vi "FPGA_PPG_reset.vi"(0 "resource_in":refnum<visa-resource-name>, 5 "error in (no error)":errorcluster) -> (14 "resource_out":refnum<visa-resource-name>, 19 "error out":errorcluster)   [LabVIEW 2014, in "NI-FPGA_PPG_Driver.lvlib"]
doc: "Resets the FPGA to default state (uninitialised).\n\nContact: Falk Ziegler, eMail: ziegler@physik.uni-greifswald.de"
uses:
  NI-FPGA_PPG_Driver.lvlib
  <vilib>/rvi/interface/nirviReadWriteControl/nirviReadWriteControl.xnode
  target/FPGA_target_state_type.ctl
  FPGA_PPG_action_type.ctl
  <vilib>/rvi/errors/niLvFpgaAdjustHostInterfaceError.vi
  FPGA_PPG_vi_ref.ctl
  FPGA Bitfiles/TiTaProj_COF_PPG_100MHz.lvbitx
  <vilib>/rvi/errors/niLvFpgaMergeErrorWithErrorCode.vi
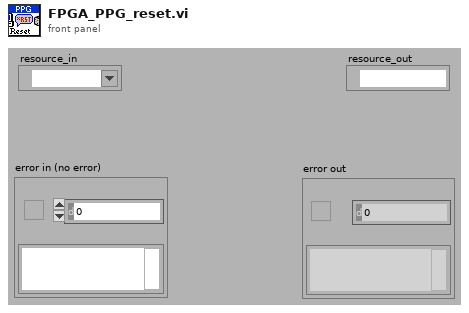
[diagram p1: front panel]
types:
  T1 = typedef "NI-FPGA_PPG_Driver.lvlib/FPGA_PPG_action_type.ctl" = enum16{"GET", "SET", "REMOVE"}
  T2 = typedef "NI-FPGA_PPG_Driver.lvlib/FPGA_PPG_vi_ref.ctl" = refnum<k20>
  T3 = typedef "NI-FPGA_PPG_Driver.lvlib/FPGA_target_state_type.ctl" = enum16{"idle", "reset", "query", "load", "run", "stopped"}
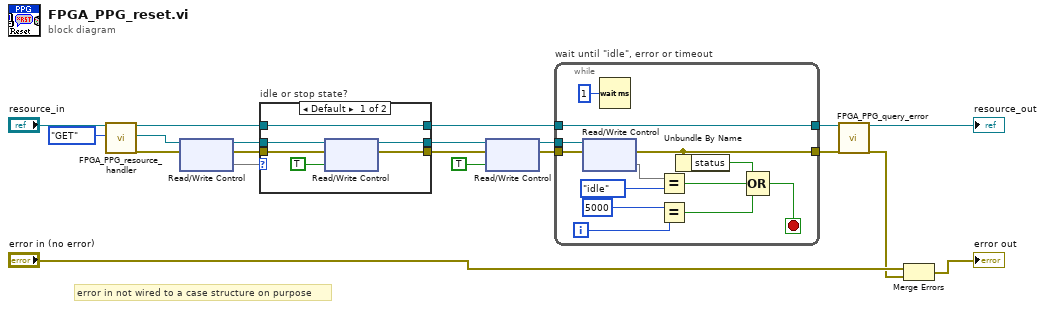
[diagram p0: block diagram]
diagram:
  # "error in not wired to a case structure on purpose"
  n1 = call "FPGA_PPG_resource_handler.vi"("resource_in"="resource_in", "action"=FPGA_PPG_action_type."GET") -> ("resource_out"=w9:refnum<visa-resource-name>, "FPGA VI Reference Out"=w11:T2, "error out"=w19:errorcluster)  [unwired: 15 in]
  n2 = xnode "Read/Write Control"("FPGA VI Reference In"=w11, "error in"=w19) -> ("FPGA VI Reference Out"=w18:T2, "error out"=w17:errorcluster, "state"=w12)
  n3 = case "idle or stop state?" shown="Default" w12 {
    tunnel: w18 -> [w26 w29]
    tunnel: w17 -> [w25 w28]
    tunnel: [w23 w29] -> w16
    tunnel: [w22 w28] -> w15
    tunnel: [w21 w27] -> w6
    tunnel: w9 -> [w21 w27]
    frame Default {
      n4 = xnode "Read/Write Control"("FPGA VI Reference In"=w26, "error in"=w25, "stop"=TRUE) -> ("FPGA VI Reference Out"=w23:T2, "error out"=w22:errorcluster)
    }
    frame "idle", "stopped" {
    }
  }
  n5 = xnode "Read/Write Control"("FPGA VI Reference In"=w16, "error in"=w15, "reset"=TRUE) -> ("FPGA VI Reference Out"=w8:T2, "error out"=w7:errorcluster)
  n6 = while "wait until \"idle\", error or timeout" {
    tunnel: w8 -> [w41]
    tunnel: w7 -> [w40]
    tunnel: w6 -> [w32]
    tunnel: [w32] -> w5
    tunnel: [w31] -> w1
    i -> [w36]
    stop <- w33 stop-if-true
    n7 = xnode "Read/Write Control"("FPGA VI Reference In"=w41, "error in"=w40) -> ("error out"=w31:errorcluster, "state"=w30)  [unwired: 1 out]
    n8 = Wait (ms)(milliseconds to wait=u32 1) -> ()  [unwired: 1 out]
    n9 = Equal?(x=w30, y=FPGA_target_state_type."idle") -> (x = y?=w37:bool)
    n10 = Equal?(x=5000, y=w36) -> (x = y?=w34:bool)
    n11 = Unbundle By Name(w31) -> ("status"=w38:bool)
    n12 = Compound Arithmetic op=OR(w38, w37, w34) -> (w33:bool)
  }
  n13 = call "FPGA_PPG_query_error.vi"("resource_in"=w5, "error in (no error)"=w1) -> ("resource_out"=→"resource_out":refnum<visa-resource-name>, "error out"=w2:errorcluster)  [unwired: 16 in]
  n14 = Merge Errors("error in (no error)", w2) -> (→"error out":errorcluster)
